vi "CSDB_Transfer.write ini.vi"(4 "error in":errorcluster, 6 "db2ini data":string[][](array[string]), 7 "db2ini instances":string[][](array[string])) -> (0 "error out":errorcluster)   [LabVIEW 2014, in "CSDB_Transfer.lvlib"]
doc: "Writes data to an inifile. The data has to be given in 2 tables :\ninstances : instancenames classnames\ndata : instancenames attributenames values"
uses:
  CSDB_Transfer.lvlib
  <vilib>/Utility/config.llb/Write Key (String).vi
  <vilib>/Utility/config.llb/NI_LVConfig.lvlib
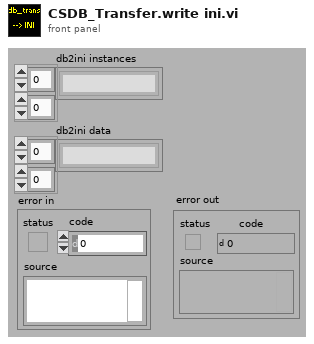
[diagram p1: front panel]
types:
  T1 = typedef "NI_LVConfig.lvlib/Config Data RefNum.ctl" = refnum<k1>
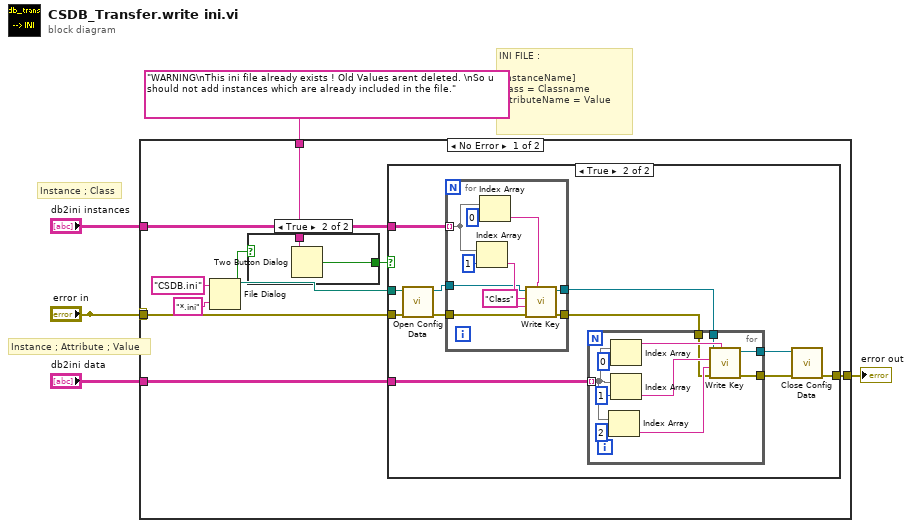
[diagram p0: block diagram]
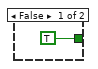
[diagram p3: hidden frame]
diagram:
  # "Instance ; Attribute ; Value"
  # "Instance ; Class"
  # "INI FILE :\n\n[InstanceName]\nClass = Classname\nAttributeName = Value"
  n1 = case shown="No Error" "error in" {
    selector: "error in" -> [_ w52]
    tunnel: [w15 w52] -> w5
    tunnel: "WARNING\nThis ini file already exists ! Old Values arent deleted. \nSo u should not add instances which are already included in the file." ("message") -> [w11 _]
    tunnel: "db2ini data" -> [w8 _]
    tunnel: "db2ini instances" -> [w7 _]
    tunnel: "error in" -> [w6 _]
    frame No Error {
      n2 = File Dialog(6:"*.ini" ("pattern"), 9:"CSDB.ini" ("default name")) -> (2:w10:bool, 3:w14:path)  [unwired: 5 in, 2 out]
      n3 = case shown="True" w10 {
        tunnel: w11 -> [_ w51]
        tunnel: [TRUE ("T button?") w50] -> w9
        frame False {
        }
        frame True {
          n4 = Two Button Dialog(message=w51) -> (T button?=w50:bool)  [unwired: 2 in]
        }
      }
      n5 = case shown="True" w9 {
        tunnel: w6 -> [w16 w27]
        tunnel: w7 -> [_ w26]
        tunnel: [w16 w23] -> w15
        tunnel: w8 -> [_ w22]
        tunnel: w14 -> [_ w17]
        frame False {
        }
        frame True {
          n6 = call <vilib>:"Open Config Data.vi"("error in (no error)"=w27, "configuration file path"=w17) -> ("error out"=w24:errorcluster, "refnum"=w25:T1)  [unwired: 7 in, 1 out]
          n7 = for {
            tunnel: w26 -> [w48] mode=indexing
            tunnel: w25 -> [w42]
            tunnel: w24 -> [w41]
            tunnel: [w40] -> w20
            tunnel: [w39] -> w21
            n8 = Index Array(array=w48, index=1) -> (element=w44:string)
            n9 = Index Array(array=w48, index=0) -> (element=w45:string)
            n10 = call-poly <vilib>:"Write Key.vi"("section"=w45, "error in (no error)"=w41, "value"=w44, "key"="Class", "refnum"=w42) -> ("error out"=w39:errorcluster, "refnum out"=w40:T1)  [unwired: 4 in, 1 out]
          }
          n11 = for {
            tunnel: w22 -> [w35] mode=indexing
            tunnel: w21 -> [w31]
            tunnel: w20 -> [w30]
            tunnel: [w29] -> w19
            tunnel: [w28] -> w18
            n12 = Index Array(array=w35, index=2) -> (element=w32:string)
            n13 = Index Array(array=w35, index=0) -> (element=w34:string)
            n14 = Index Array(array=w35, index=1) -> (element=w33:string)
            n15 = call-poly <vilib>:"Write Key.vi"("section"=w34, "error in (no error)"=w31, "value"=w32, "key"=w33, "refnum"=w30) -> ("error out"=w28:errorcluster, "refnum out"=w29:T1)  [unwired: 4 in, 1 out]
          }
          n16 = call <vilib>:"Close Config Data.vi"("error in (no error)"=w18, "refnum"=w19) -> ("error out"=w23:errorcluster)  [unwired: 8 in, 1 out]
        }
      }
    }
    frame Error {
    }
  }
  "error out" <- w5
